vi "GenerationConfig.vi"() -> ()   [LabVIEW 2025]
uses:
  <vilib>/DAQmx/create/channels.llb/DAQmx Create Channel (AO-Voltage-Basic).vi
  <vilib>/DAQmx/configure/timing.llb/DAQmx Timing (Use Waveform).vi
panel:
  out "error out":errorcluster
  out "task out":refnum<k21>
  out "number of samples":dbl
  in  "frequency settings":T1={"frequency (Hz)"=0.001, "number of samples per cycle"=2.0, "number of cycles"=1.0} {"frequency (Hz)" min=0.001 max=100000000.0; "number of samples per cycle" min=2.0 step=1.0; "number of cycles" min=1.0}
  in  "error in":errorcluster
  in  "physical channels":tag
  in  "channel settings":T2={"units"=10348, "input terminal configuration"=-1, "minimum value"=-5.0, "maximum value"=5.0} {"units" items=["Volts"=10348, "From Custom Scale"=10065]; "input terminal configuration" items=["Default"=-1, "RSE"=10083, "NRSE"=10078, "Differential"=10106, "Pseudodifferential"=12529]}
  # "Configuración de la DAQ para\ngeneración de datos"
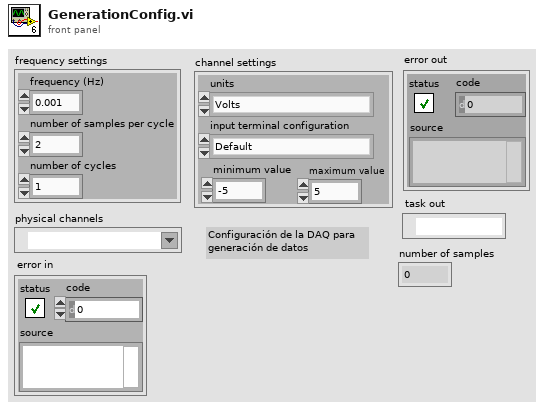
[diagram p1: front panel]
types:
  T1 = cluster{"frequency (Hz)":dbl, "number of samples per cycle":dbl, "number of cycles":dbl}
  T2 = cluster{"units":i32, "input terminal configuration":i32, "minimum value":dbl, "maximum value":dbl}
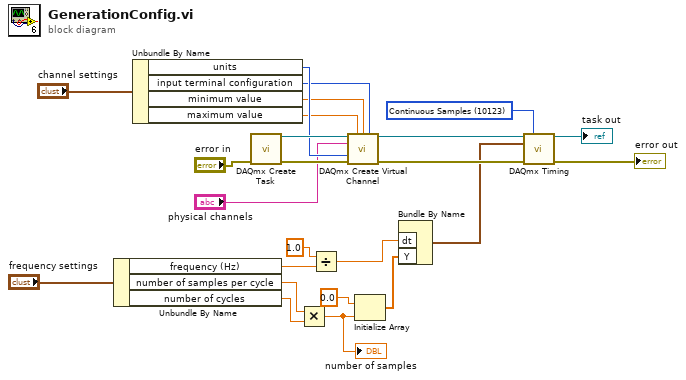
[diagram p0: block diagram]
diagram:
  w15 = 10123 items=["Finite Samples"=10178, "Continuous Samples"=10123, "Hardware Timed Single Point"=12522] ("sample mode")
  n1 = Unbundle By Name("frequency settings") -> ("frequency (Hz)"=w11:dbl, "number of samples per cycle"=w10:dbl, "number of cycles"=w9:dbl)
  n2 = Unbundle By Name("channel settings") -> ("units"=w21:i32, "input terminal configuration"=w20:i32, "minimum value"=w19:dbl, "maximum value"=w18:dbl)
  n3 = call <vilib>:"DAQmx Create Task.vi"("error in"="error in") -> ("task out"=w24:refnum<k21>, "error out"=w23:errorcluster)  [unwired: 13 in]
  n4 = Multiply(x=w10, y=w9) -> (x*y=w3:dbl)
  "number of samples" <- w3
  n5 = Divide(x=1.0, y=w11) -> (x/y=w14:dbl)
  n6 = call-poly <vilib>:"DAQmx Create Virtual Channel.vi"("task in"=w24, "maximum value"=w18, "minimum value"=w19, "output terminal configuration"=w20, "physical channels"="physical channels", "units"=w21, "error in"=w23) -> ("task out"=w5:refnum<k21>, "error out"=w6:errorcluster)  [unwired: 7 in]
  n7 = Initialize Array(0.0 ("element"), w3) -> (w7:dbl[])
  n8 = Bundle By Name("dt"=w14, "Y"=w7) -> (w4:waveform(dbl))  [unwired: 1 in]
  n9 = call-poly <vilib>:"DAQmx Timing.vi"("task/channels in"=w5, "sample mode"=w15, "waveform"=w4, "error in"=w6) -> ("task out"=→"task out":refnum<k21>, "error out"=→"error out":errorcluster)  [unwired: 10 in]
